vi "XLP80_CAN_MaskBytes_GetDBC_Values.vi"() -> ()   [LabVIEW 2021]
uses:
  <vilib>/xnet/xnet.llb/XNET Database Close (Signal).vi
  <vilib>/xnet/xnet.llb/XNET Database Close (Cluster).vi
  <resource>/objmgr/xnet.rc
panel:
  out "MuxDynamic":bool[](array[boolean])
  out "Mux":bool[](array[boolean])
  out "DBC Settings":T1={"ByteOrder"=[enum."Motorola", enum."Motorola"], "Type"=[], "Factor"=[1.0, 1.0], "Offset"=[0.0, 0.0], "Startbit"=[27, 43], "Length"=[16, 16], "Mux"=[FALSE, FALSE], "Name"=["", ""]} {"Offset" format="%.3f"; "Factor" format="%.3f"}
  in  "default baud rate (0)":u64=500000
  in  "CAN DBC":path=path "G:/07_GLOBE/00_git/XLP80/02_Documentation/Daten Albert_10-08-2022/Globe_CAN_500_2022-08-08_v26.dbc"
  out "Frame":string[](array[string])
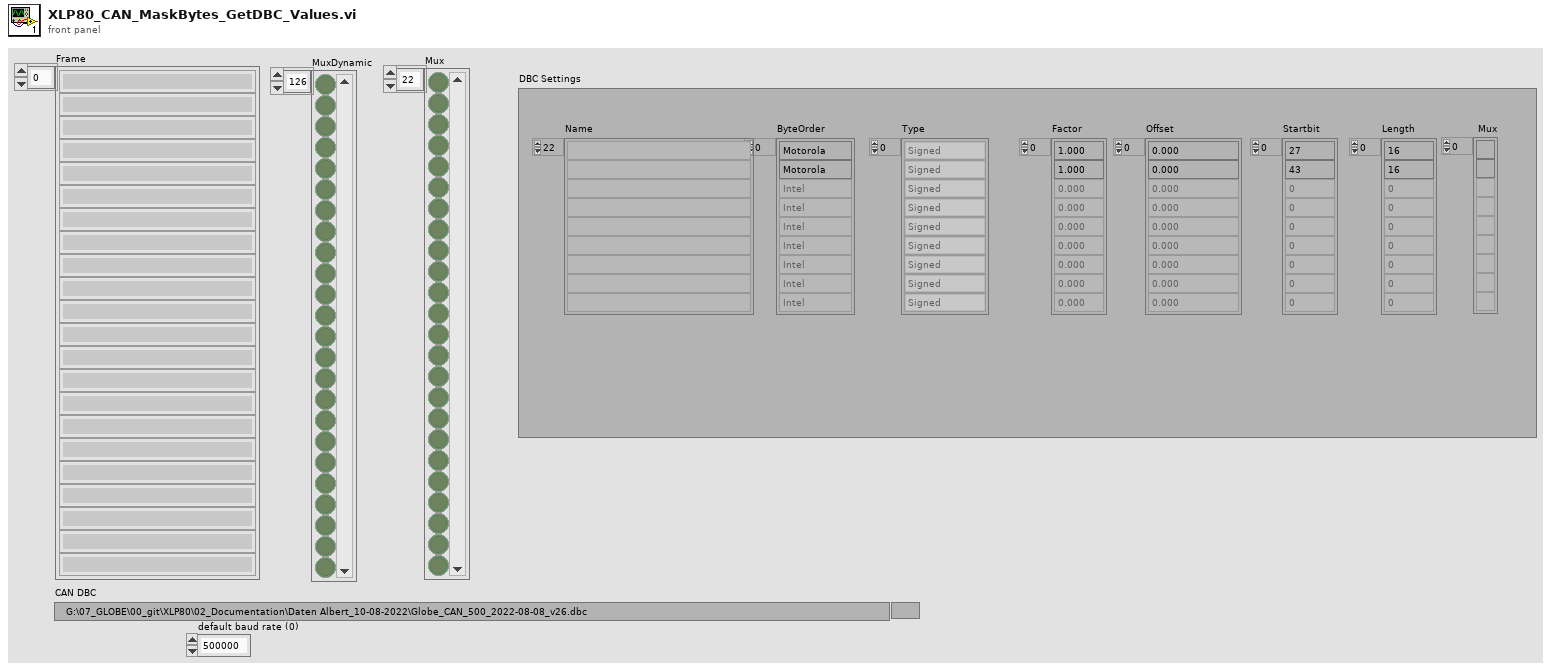
[diagram p1: front panel]
types:
  T1 = cluster{"ByteOrder":enum16{"Intel", "Motorola"}[], "Type":enum16{"Signed", "Unsigned", "IEEE Float", "Byte Array"}[], "Factor":dbl[], "Offset":dbl[], "Startbit":u32[], "Length":u32[], "Mux":bool[], "Name":string[]}
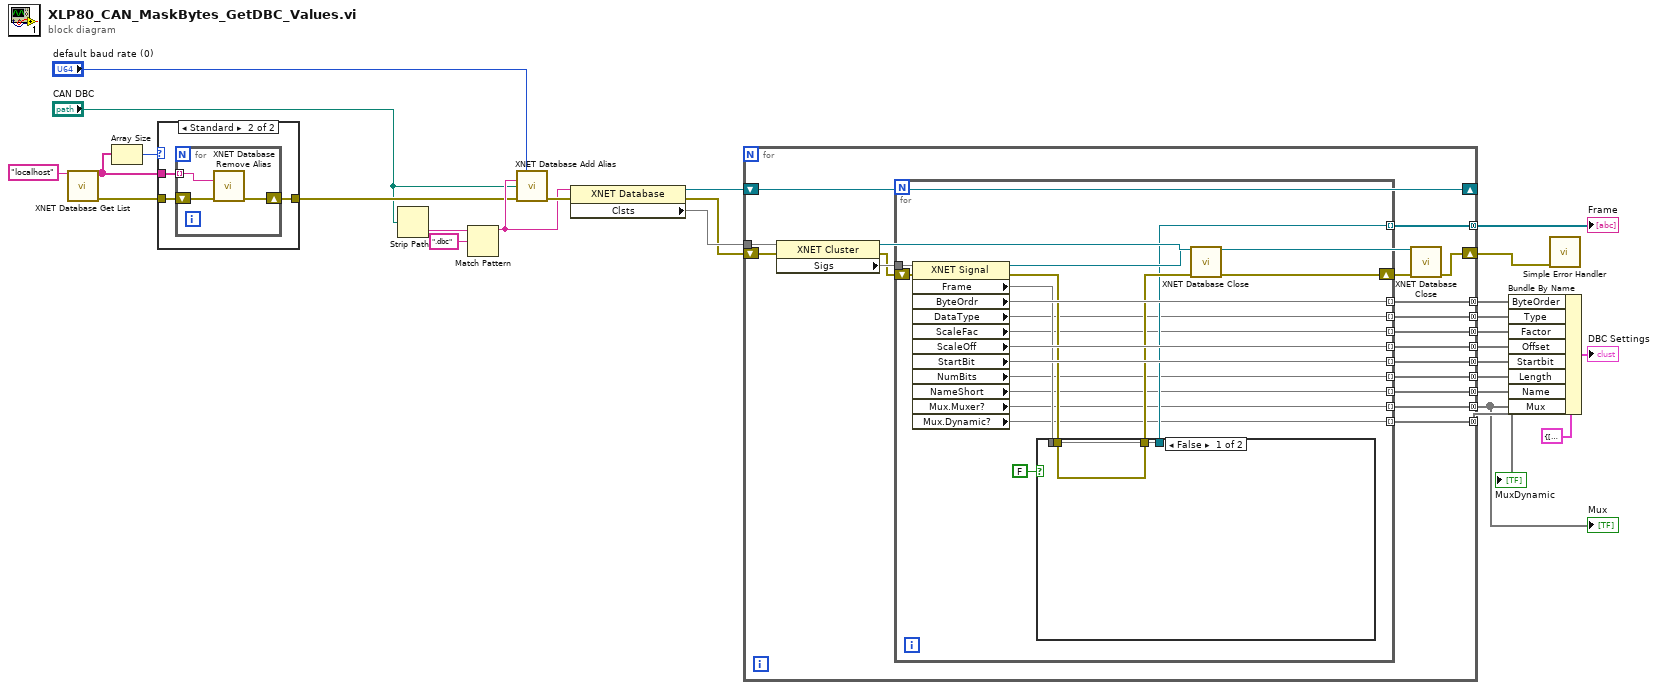
[diagram p0: block diagram]
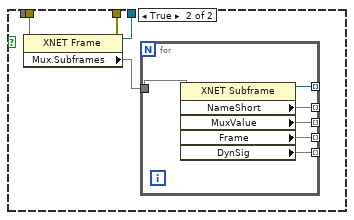
[diagram p3: hidden frame]
diagram:
  n1 = call <vilib>:"XNET Database Get List.vi"("IP address (localhost)"="localhost") -> ("array of alias"=w17:string[], "error out"=w19:errorcluster)  [unwired: 12 in, 1 out]
  n2 = Array Size(array=w17) -> (size(s)=w16:i32)
  n3 = case shown="Standard" w16 {
    tunnel: w19 -> [w28 w31]
    tunnel: [w28 w30] -> w18
    tunnel: w17 -> [_ w29]
    frame 0 {
    }
    frame Default {
      n4 = for {
        shift-right: [w33] -> w30
        shift-left: w31 -> [w34]
        tunnel: w29 -> [w32] mode=indexing
        n5 = call <vilib>:"XNET Database Remove Alias.vi"("alias"=w32, "error in (no error)"=w34) -> ("error out"=w33:errorcluster)  [unwired: 13 in]
      }
    }
  }
  n6 = Strip Path(path="CAN DBC") -> (name=w22:string)  [unwired: 1 out]
  n7 = Match Pattern(string=w22, regular expression=".dbc") -> (before substring=w21:string)  [unwired: 1 in, 3 out]
  n8 = call <vilib>:"XNET Database Add Alias.vi"("default baud rate (0)"="default baud rate (0)", "alias"=w21, "filepath"="CAN DBC", "error in (no error)"=w18) -> ("error out"=w24:errorcluster)  [unwired: 11 in]
  n9 = property class="XNET Database"(reference=w21, error in=w24) -> (reference out=w26:refnum<k21>, error out=w15:errorcluster, "Clsts"=w27)
  n10 = for {
    tunnel: w27 -> [w52]
    shift-right: [w45] -> _
    shift-left: w26 -> [w45]
    tunnel: [w50] -> w5 mode=concatenating
    tunnel: [w49] -> w6 mode=concatenating
    tunnel: [w48] -> w8 mode=concatenating
    tunnel: [w47] -> w25 mode=concatenating
    tunnel: [w46] -> w9 mode=concatenating
    shift-right: [w42] -> w14
    shift-left: w15 -> [w44]
    tunnel: [w39] -> w4 mode=concatenating
    tunnel: [w38] -> w10 mode=concatenating
    tunnel: [w37] -> w7 mode=concatenating
    tunnel: [w36] -> w3 mode=concatenating
    tunnel: [w35] -> w1 mode=concatenating
    n11 = property class="XNET Cluster"(reference=w52, error in=w44) -> (reference out=w43:refnum<k21>, error out=w41:errorcluster, "Sigs"=w51)
    n12 = for {
      tunnel: w51 -> [w70]
      tunnel: [w69] -> w50 mode=indexing
      tunnel: [w68] -> w49 mode=indexing
      tunnel: [w56] -> w48 mode=indexing
      tunnel: [w60] -> w47 mode=indexing
      tunnel: [w64] -> w46 mode=indexing
      shift-right: [w66] -> w40
      shift-left: w41 -> [w67]
      tunnel: [w59] -> w39 mode=indexing
      tunnel: [w57] -> w38 mode=indexing
      tunnel: [w55] -> w37 mode=indexing
      tunnel: [w54] -> w36 mode=indexing
      tunnel: [w53] -> w35 mode=indexing
      n13 = property class="XNET Signal"(reference=w70, error in=w67) -> (reference out=w65:refnum<k21>, error out=w62:errorcluster, "Frame"=w63, "ByteOrdr"=w64, "DataType"=w56, "ScaleFac"=w55, "ScaleOff"=w68, "StartBit"=w69, "NumBits"=w59, "NameShort"=w54, "Mux.Muxer?"=w53, "Mux.Dynamic?"=w57)
      n14 = case shown="False" FALSE {
        tunnel: w63 -> [w71 w77]
        tunnel: [w71 w74] -> w60
        tunnel: w62 -> [w72 w76]
        tunnel: [w72 w75] -> w61
        frame False {
        }
        frame True {
          n15 = property class="XNET Frame"(reference=w77, error in=w76) -> (reference out=w74:refnum<k21>, error out=w75:errorcluster, "Mux.Subframes"=w73)
          n16 = for {
            tunnel: w73 -> [w83]
            tunnel: [w82] -> _ mode=indexing
            tunnel: [w81] -> _ mode=indexing
            tunnel: [w80] -> _ mode=indexing
            tunnel: [w79] -> _ mode=indexing
            tunnel: [w78] -> _ mode=indexing
            n17 = property class="XNET Subframe"(reference=w83) -> (reference out=w78:refnum<k21>, "NameShort"=w82, "MuxValue"=w81, "Frame"=w80, "DynSig"=w79)  [unwired: 1 in, 1 out]
          }
        }
      }
      n18 = call-poly <vilib>:"XNET Database Close.vi"("signal in"=w65, "error in (no error)"=w61) -> ("error out"=w66:errorcluster)  [unwired: 13 in]
    }
    n19 = call-poly <vilib>:"XNET Database Close.vi"("cluster in"=w43, "error in (no error)"=w40) -> ("error out"=w42:errorcluster)  [unwired: 13 in]
  }
  "Frame" <- w25
  "Mux" <- w1
  "MuxDynamic" <- w10
  n20 = Bundle By Name(cluster=T1 {"ByteOrder"=[], "Type"=[], "Factor"=[], "Offset"=[], "Startbit"=[], "Length"=[], "Mux"=[], "Name"=[]} ("DBC Settings"), "ByteOrder"=w9, "Type"=w8, "Factor"=w7, "Offset"=w6, "Startbit"=w5, "Length"=w4, "Name"=w3, "Mux"=w1) -> (→"DBC Settings":T1)
  n21 = call <vilib>:"Simple Error Handler.vi"("error in (no error)"=w14) -> ()  [unwired: 4 in, 5 out]
